vi "Create Locks.vi"(8 "error in (no error)":errorcluster, 11 "WebSocket Client in":refnum<class "WebSocket Client.lvclass">) -> (0 "error out":errorcluster, 3 "WebSocket Client out":refnum<class "WebSocket Client.lvclass">)   [LabVIEW 2020, in "HTTP Server.lvlib" / "WebSocket Client.lvclass"]
uses:
  WebSocket Client.lvclass
  WebSocket Client.lvclass/WebSocket Client.ctl
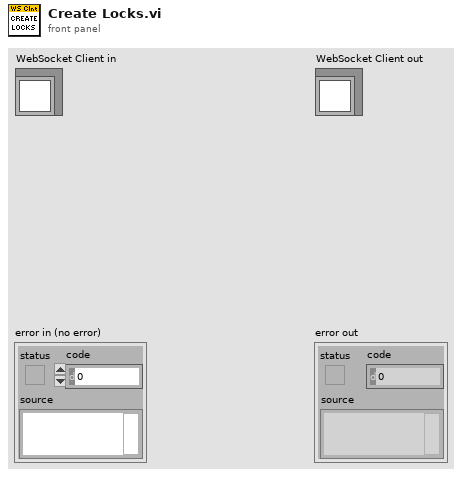
[diagram p1: front panel]
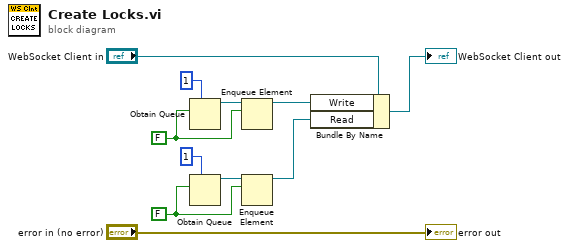
[diagram p0: block diagram]
diagram:
  w6 = FALSE
  w7 = FALSE
  n1 = Obtain Queue(max queue size (-1, unlimited)=1, element data type=w7) -> (queue out=w8:refnum<queue>)  [unwired: 3 in, 2 out]
  n2 = Obtain Queue(max queue size (-1, unlimited)=1, element data type=w6) -> (queue out=w5:refnum<queue>)  [unwired: 3 in, 2 out]
  n3 = Enqueue Element(queue=w8, element=w7) -> (queue out=w2:refnum<queue>)  [unwired: 2 in, 2 out]
  n4 = Enqueue Element(queue=w5, element=w6) -> (queue out=w1:refnum<queue>)  [unwired: 2 in, 2 out]
  n5 = Bundle By Name(cluster="WebSocket Client in", "Write"=w2, "Read"=w1) -> (→"WebSocket Client out":refnum<class "WebSocket Client.lvclass">)
  "error out" <- "error in (no error)"
